vi "Connection Callback.vi"(7 "Owner":refnum<class>, 8 "error in (no error)":errorcluster, 9 "Context":variant, 10 "Connection State":T1, 11 "Connection":refnum<class "Connection.lvclass">) -> (0 "error out":errorcluster)   [LabVIEW 2020, in "PicoG-Core.lvlib" / "Resource.lvclass"]
uses:
  Resource.lvclass
  Resource.lvclass/Resource.ctl
  <vilib>/IlluminatedG/lv-stream/Connection/Connection.lvclass
  <vilib>/IlluminatedG/lv-stream/stream/Stream.lvclass
  <vilib>/IlluminatedG/lv-stream/Connection State.ctl
  <vilib>/IlluminatedG/lv-stream/Stream.lvlib
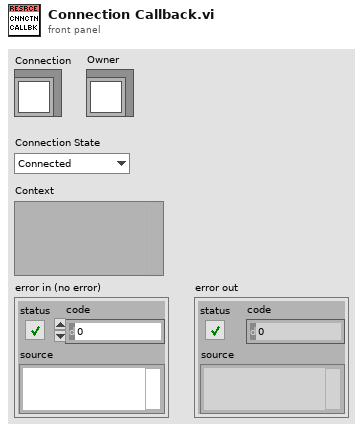
[diagram p1: front panel]
types:
  T1 = typedef "Stream.lvlib/Connection State.ctl" = enum16{"Connected", "Disconnected"}
  T2 = typedef "PicoG-Core.lvlib/Resource.lvclass/Ref Data.ctl" = cluster{"Config":map{string, string}, "Connection":refnum<class "Connection.lvclass">, "Stream":refnum<class "Stream.lvclass">}
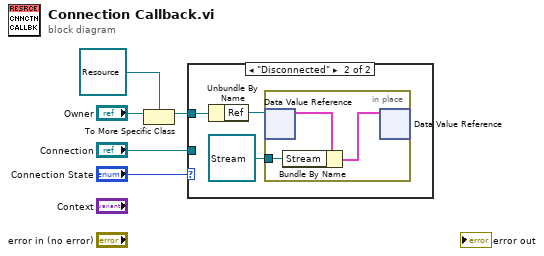
[diagram p0: block diagram]
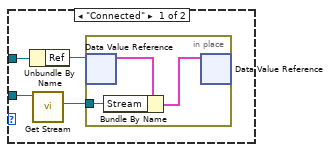
[diagram p2: hidden frame]
diagram:
  n1 = To More Specific Class(target class=refnum<class "Resource.lvclass"> refnum ("PicoG-Core:Resource"), reference="Owner") -> (specific class reference=w1:refnum<class "Resource.lvclass">)  [unwired: 1 in, 1 out]
  n2 = case shown="\"Disconnected\"" "Connection State" {
    tunnel: "Connection" -> [w9 _]
    tunnel: w1 -> [w8 w15]
    frame "Connected" {
      n3 = Unbundle By Name(w8) -> ("Ref"=w7:refnum<data-value>)
      n4 = call-dynamic "Get Stream.vi"("Connection in"=w9) -> ("Stream"=w6:refnum<class "Stream.lvclass">)  [unwired: 8 in, 2 out]
      n5 = in-place {
        in-place-border: w6 -> [w11]
        n6 = in-place-dvr #1(w7) -> (w12:T2)  [unwired: 1 out]
        n7 = Bundle By Name(cluster=w12, "Stream"=w11) -> (w10:T2)
        n8 = in-place-dvr #1(w10) -> ()  [unwired: 2 out]
      }
    }
    frame "Disconnected" {
      n9 = Unbundle By Name(w15) -> ("Ref"=w14:refnum<data-value>)
      n10 = in-place {
        in-place-border: refnum<class "Stream.lvclass"> refnum ("Stream") -> [w17]
        n11 = in-place-dvr #2(w14) -> (w18:T2)  [unwired: 1 out]
        n12 = Bundle By Name(cluster=w18, "Stream"=w17) -> (w16:T2)
        n13 = in-place-dvr #2(w16) -> ()  [unwired: 2 out]
      }
    }
  }
